vi "Result_Test.vi"(8 "error in (no error)":errorcluster caption="entrée d'erreur (pas d'erreur)", 11 "Get_Voltage en entrée":refnum<class "P2056_Set_SN.lvclass">) -> (0 "error out":errorcluster caption="sortie d'erreur", 3 "Get_Voltage en sortie":refnum<class "P2056_Set_SN.lvclass">)   [LabVIEW 2020, in "Library Test.lvlib" / "P2056_Set_SN.lvclass"]
uses:
  P2056_Set_SN.lvclass
  C:/Users/ngarcin/OneDrive - Altyor/Standard TB/Class/Test/Test (Default)/Test (Default).lvclass
  JSON API/JSON Value/Set from JSON string.vi
  JSON API/JSON Value/JSON Value.lvclass
  P2056_Send_Command_UART.lvclass
  P2056_Set_SN.lvclass/P2056_Set_SN.ctl
  JSON API/Variant JSON/Variant JSON.lvlib
  JSON API/Get Polymorphic/JSON GetSet.lvlib
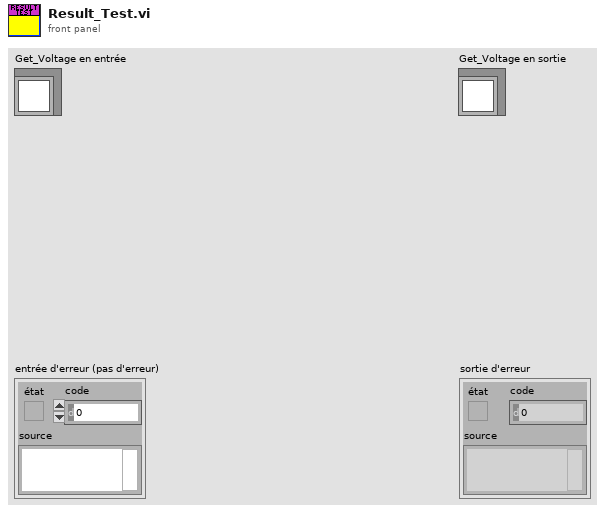
[diagram p1: front panel]
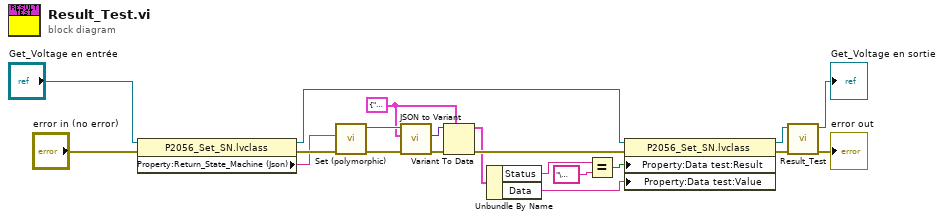
[diagram p0: block diagram]
diagram:
  w13 = cluster{"Data":string, "Status":string} {"Data"="", "Status"=""}
  n1 = property class="P2056_Set_SN.lvclass"(reference="Get_Voltage en entrée", error in="error in (no error)") -> (reference out=w18:refnum<class "P2056_Set_SN.lvclass">, error out=w12:errorcluster, "Property:Return_State_Machine (Json)"=w10:string)
  n2 = call-poly "Set (polymorphic).vi"("error in (no error)"=w12, "JSON stream"=w10) -> ("error out"=w15:errorcluster, "JSON Value out"=w17:refnum<class "JSON Value.lvclass">)  [unwired: 7 in, 1 out]
  n3 = call "JSON to Variant.vi"("error in (no error)"=w15, "Variant (Data Type)"=w13, "JSON Value"=w17) -> ("error out"=w16:errorcluster, "Variant out"=w14:variant)  [unwired: 7 in]
  n4 = Variant To Data(error in=w16, type=w13, Variant=w14) -> (data=w9:cluster{"Data":string, "Status":string}, error out=w11:errorcluster)
  n5 = Unbundle By Name(w9) -> ("Status"=w8:string, "Data"=w5:string)
  n6 = Equal?(x=w8, y="\u0000") -> (x = y?=w6:bool)
  n7 = property class="P2056_Set_SN.lvclass"(reference=w18, error in=w11, "Property:Data test:Result"=w6, "Property:Data test:Value"=w5) -> (reference out=w2:refnum<class "P2056_Set_SN.lvclass">, error out=w1:errorcluster)
  n8 = call-parent "Result_Test.vi"("error in (no error)"=w1, "Get_Voltage en entrée"=w2) -> ("error out"=→"error out":errorcluster, "Get_Voltage en sortie"=→"Get_Voltage en sortie":refnum<class "P2056_Set_SN.lvclass">)  [unwired: 8 in]
